vi "ImageOverlay.vi"(7 "RGB_Image":T2, 8 "Error In":errorcluster, 9 "Overlay?":bool, 10 "UI Controls Refnum":T3, 11 "Image Input Cluster":T1) -> (0 "Error Out":errorcluster, 3 "Saved Image":T2)   [LabVIEW 2012]
uses:
  <vilib>/vision/Image Controls.llb/IMAQ Image.ctl
  Custom Control and Typedefs/UI Controls Refnum.ctl
  Custom Control and Typedefs/ChannelSelector_for_PosSave.ctl
  Custom Controls/PositionSaveMod.ctl
  Custom Control and Typedefs/Overlay Control.ctl
  Custom Control and Typedefs/ImageCluster.ctl
  <vilib>/vision/NI_Vision_Development_Module.lvlib
panel:
  # "Red (Current Image)"
  # "Green (Saved Image)"
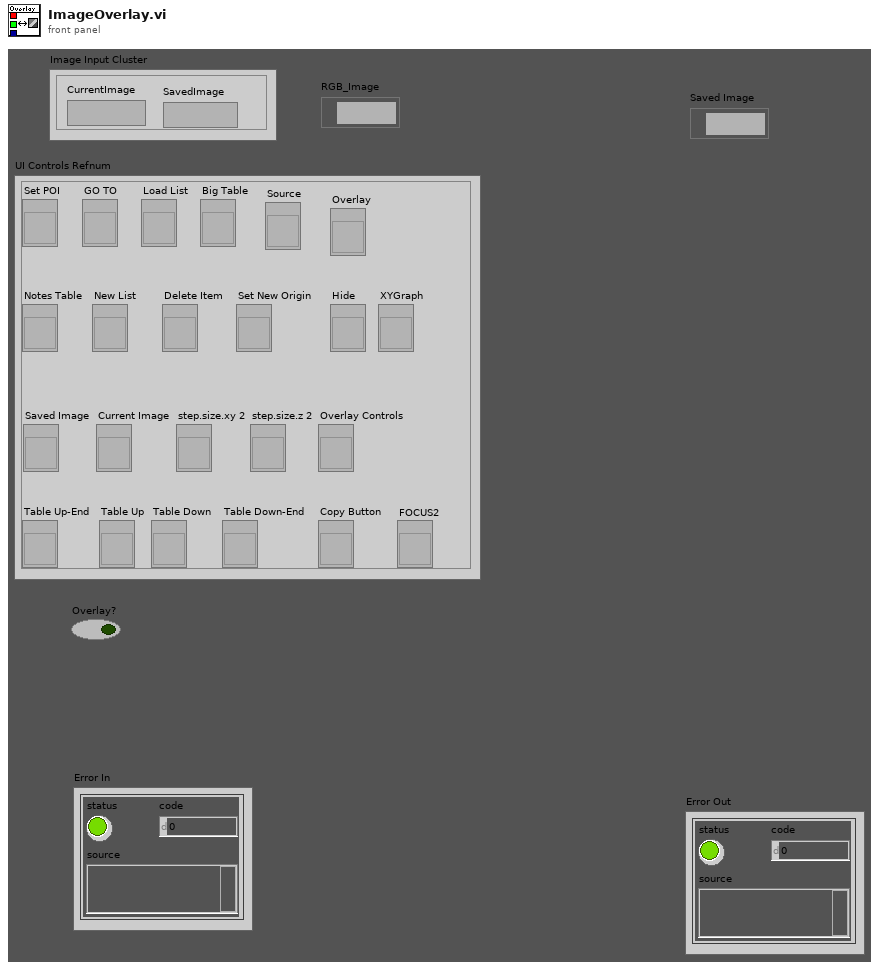
[diagram p1: front panel]
types:
  T1 = typedef "ImageCluster.ctl" = cluster{"CurrentImage":T2, "SavedImage":T2}
  T2 = typedef "IMAQ Image.ctl" = refnum<image>
  T3 = typedef "UI Controls Refnum.ctl" = cluster{"GO TO":refnum<vi>, "Load List":refnum<vi>, "Big Table":refnum<vi>, "Notes Table":refnum<vi>, "New List":refnum<vi>, "Delete Item":refnum<vi>, "Set New Origin":refnum<vi>, "Set POI":refnum<vi>, "Saved Image":refnum<vi>, "Current Image":refnum<vi>, "step.size.xy 2":refnum<vi>, "step.size.z 2":refnum<vi>, "Source":refnum<vi>, "Table Up-End":refnum<vi>, "Table Up":refnum<vi>, "Table Down":refnum<vi>, "Table Down-End":refnum<vi>, "Copy Button":refnum<vi>, "Hide":refnum<vi>, "Overlay Controls":refnum<vi>, "Overlay":refnum<vi>, "XYGraph":refnum<vi>, "FOCUS2":refnum<vi>}
  T4 = typedef "Overlay Control.ctl" = cluster{"auto scale\n      Red ":bool, "Min Max Saved (Green)":cluster{dbl, dbl}, "auto scale\n      Green":bool, "Min Max Saved (Red)":cluster{dbl, dbl}}
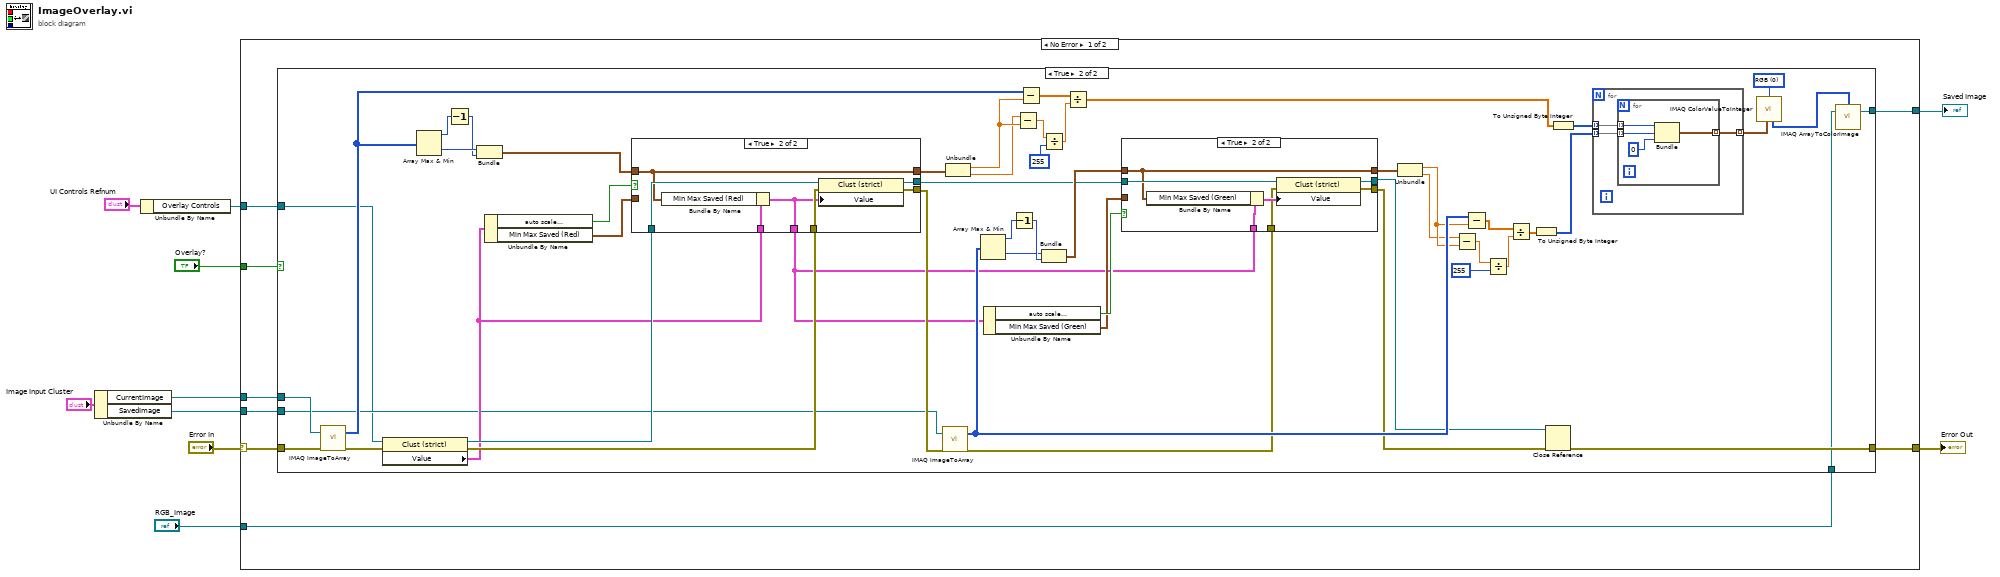
[diagram p0: block diagram]
diagram:
  n1 = Unbundle By Name("Image Input Cluster") -> ("CurrentImage"=w8:T2, "SavedImage"=w7:T2)
  n2 = Unbundle By Name("UI Controls Refnum") -> ("Overlay Controls"=w5:refnum<vi>)
  n3 = case shown="No Error" "Error In" {
    selector: "Error In" -> [w17 w101]
    tunnel: [w14 w101] -> w10
    tunnel: w8 -> [w18 _]
    tunnel: w7 -> [w16 w102]
    tunnel: [w15 w102] -> w6
    tunnel: w5 -> [w13 _]
    tunnel: "Overlay?" -> [w12 _]
    tunnel: "RGB_Image" -> [w11 _]
    frame No Error {
      n4 = case shown="True" w12 {
        tunnel: w18 -> [_ w57]
        tunnel: w17 -> [w19 w56]
        tunnel: w16 -> [w20 w28]
        tunnel: [w20 w27] -> w15
        tunnel: [w19 w24] -> w14
        tunnel: w13 -> [_ w23]
        tunnel: w11 -> [_ w22]
        frame False {
        }
        frame True {
          w59 = u16 0 items=["RGB", "HSL", "HSV", "HSI"] ("Color Mode")
          n5 = call "IMAQ ImageToArray"("error in (no error)"=w56, "Image"=w57) -> ("error out"=w51:errorcluster, "Image Pixels (I16)"=w52:i16[][])  [unwired: 2 in, 3 out]
          n6 = property class="Clust (strict)"(reference=w23, error in=w51) -> (reference out=w47:refnum<vi>, error out=w43:errorcluster, "Value"=w33:T4)
          n7 = Array Max & Min(array=w52) -> (max value=w55:i16, min value=w54:i16)  [unwired: 2 out]
          n8 = Decrement(x=w55) -> (x-1=w53:i16)
          n9 = Bundle(w54, w53) -> (w49:cluster{i16, i16})  [unwired: 1 in]
          n10 = Unbundle By Name(w33) -> ("auto scale\n      Red"=w50:bool, "Min Max Saved (Red)"=w48:cluster{dbl, dbl})
          n11 = case shown="True" w50 {
            tunnel: w49 -> [_ w91]
            tunnel: w48 -> [w86 _]
            tunnel: w47 -> [w84 w93]
            tunnel: w33 -> [w83 w92]
            tunnel: [w86 w91] -> w46
            tunnel: [w84 w90] -> w35
            tunnel: w43 -> [w85 w89]
            tunnel: [w85 w88] -> w42
            tunnel: [w83 w87] -> w21
            frame False {
            }
            frame True {
              n12 = Bundle By Name(cluster=w92, "Min Max Saved (Red)"=w91) -> (w87:T4)
              n13 = property class="Clust (strict)"(reference=w93, error in=w89, "Value"=w87) -> (reference out=w90:refnum<vi>, error out=w88:errorcluster)
            }
          }
          n14 = call "IMAQ ImageToArray"("error in (no error)"=w42, "Image"=w28) -> ("error out"=w32:errorcluster, "Image Pixels (I16)"=w38:i16[][])  [unwired: 2 in, 3 out]
          n15 = Unbundle(w46) -> (w45:dbl, w44:dbl)
          n16 = Array Max & Min(array=w38) -> (max value=w39:i16, min value=w40:i16)  [unwired: 2 out]
          n17 = Unbundle By Name(w21) -> ("auto scale\n      Green"=w36:bool, "Min Max Saved (Green)"=w34:cluster{dbl, dbl})
          n18 = Decrement(x=w39) -> (x-1=w41:i16)
          n19 = Subtract(x=w44, y=w45) -> (x-y=w63:dbl)
          n20 = Subtract(x=w52, y=w45) -> (x-y=w72:dbl[][])
          n21 = Bundle(w40, w41) -> (w37:cluster{i16, i16})  [unwired: 1 in]
          n22 = Divide(x=w63, y=i16 255) -> (x/y=w71:dbl)
          n23 = Divide(x=w72, y=w71) -> (x/y=w69:dbl[][])
          n24 = case shown="True" w36 {
            tunnel: w37 -> [_ w79]
            tunnel: w34 -> [w75 _]
            tunnel: w35 -> [w73 w82]
            tunnel: w21 -> [_ w81]
            tunnel: [w75 w79] -> w31
            tunnel: [w73 w78] -> w25
            tunnel: w32 -> [w74 w77]
            tunnel: [w74 w76] -> w26
            frame False {
            }
            frame True {
              n25 = Bundle By Name(cluster=w81, "Min Max Saved (Green)"=w79) -> (w80:T4)
              n26 = property class="Clust (strict)"(reference=w82, error in=w77, "Value"=w80) -> (reference out=w78:refnum<vi>, error out=w76:errorcluster)
            }
          }
          n27 = Unbundle(w31) -> (w30:dbl, w29:dbl)
          n28 = Subtract(x=w29, y=w30) -> (x-y=w64:dbl)
          n29 = Subtract(x=w38, y=w30) -> (x-y=w65:dbl[][])
          n30 = Divide(x=w64, y=i16 255) -> (x/y=w66:dbl)
          n31 = Divide(x=w65, y=w66) -> (x/y=w68:dbl[][])
          n32 = To Unsigned Byte Integer(number=w68) -> (unsigned 8bit integer=w61:u8[][])
          n33 = Close Reference(reference=w25, error in (no error)=w26) -> (error out=w24:errorcluster)
          n34 = To Unsigned Byte Integer(number=w69) -> (unsigned 8bit integer=w62:u8[][])
          n35 = for {
            tunnel: w62 -> [w95] mode=indexing
            tunnel: w61 -> [w96] mode=indexing
            tunnel: [w94] -> w60 mode=indexing
            n36 = for {
              tunnel: w96 -> [w100] mode=indexing
              tunnel: w95 -> [w99] mode=indexing
              tunnel: [w98] -> w94 mode=indexing
              n37 = Bundle(w99, w100, u8 0) -> (w98:cluster{u8, u8, u8})  [unwired: 1 in]
            }
          }
          n38 = call "IMAQ ColorValueToInteger"("2D Color value array"=w60, "Color Mode"=w59) -> ("2D U32 array"=w58:u32[][])  [unwired: 3 in, 3 out]
          n39 = call "IMAQ ArrayToColorImage"("Image Pixels (U32)"=w58, "Image"=w22) -> ("Image Out"=w27:T2)  [unwired: 3 in, 1 out]
        }
      }
    }
    frame Error {
    }
  }
  "Error Out" <- w10
  "Saved Image" <- w6
